vi "Gravity Loading.vi"   [LabVIEW 2017, in "NI_Kinematics.lvlib"]
doc: "Calculates the torque that gravity applies to each joint of a robotic arm. Wire data to the <B>joint positions</B> input to determine the polymorphic instance to use or manually select the instance. \n\n<B>.m file:</B> gravload"
uses:
  <vilib>/robotics/Kinematics/NI_Kinematics.lvlib
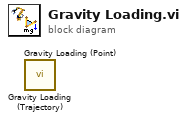
[diagram p0: block diagram]
diagram:
  n1 = call <vilib>:"Gravity Loading (Trajectory).vi"() -> ()  [unwired: 9 in, 3 out]
  n2 = call <vilib>:"Gravity Loading (Point).vi"() -> ()  [unwired: 9 in, 3 out]
